vi "pic-labview.vi"() -> ()   [LabVIEW 2020]
uses:
  <vilib>/Instr/_visa.llb/VISA Configure Serial Port (Instr).vi
  <vilib>/ErrorRing/Error Ring.xnode
panel:
  out "error out":errorcluster
  out "reference out":refnum<visa-resource-name>
  in  "Boolean 4":bool
  in  "Boolean 3":bool
  in  "Boolean 2":bool
  in  "Boolean":bool
  out "Thermometer":i32(slide) scale=0.0..1023.0
  out "value":i32
  out "read buffer":string
  in  "Puerto Serial":refnum<visa-resource-name>
  in  "stop":bool
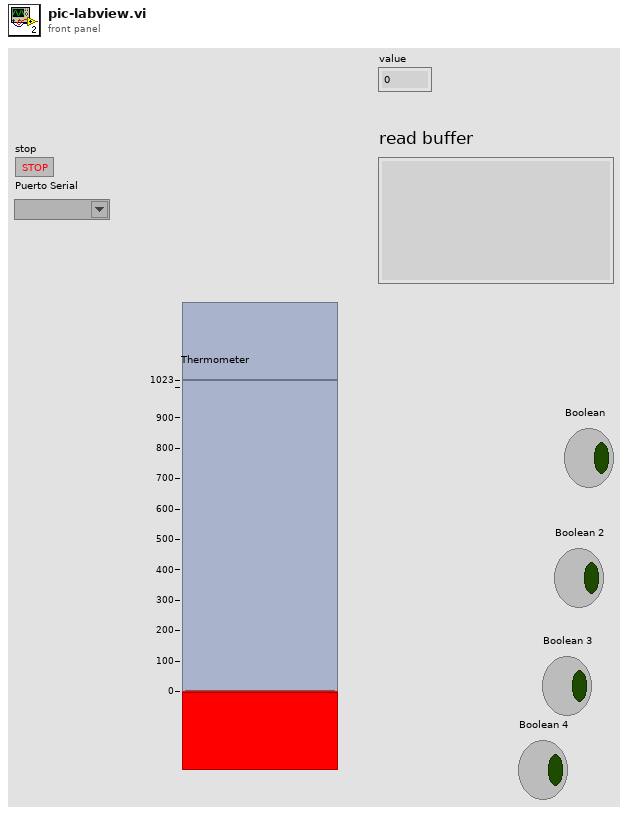
[diagram p1: front panel]
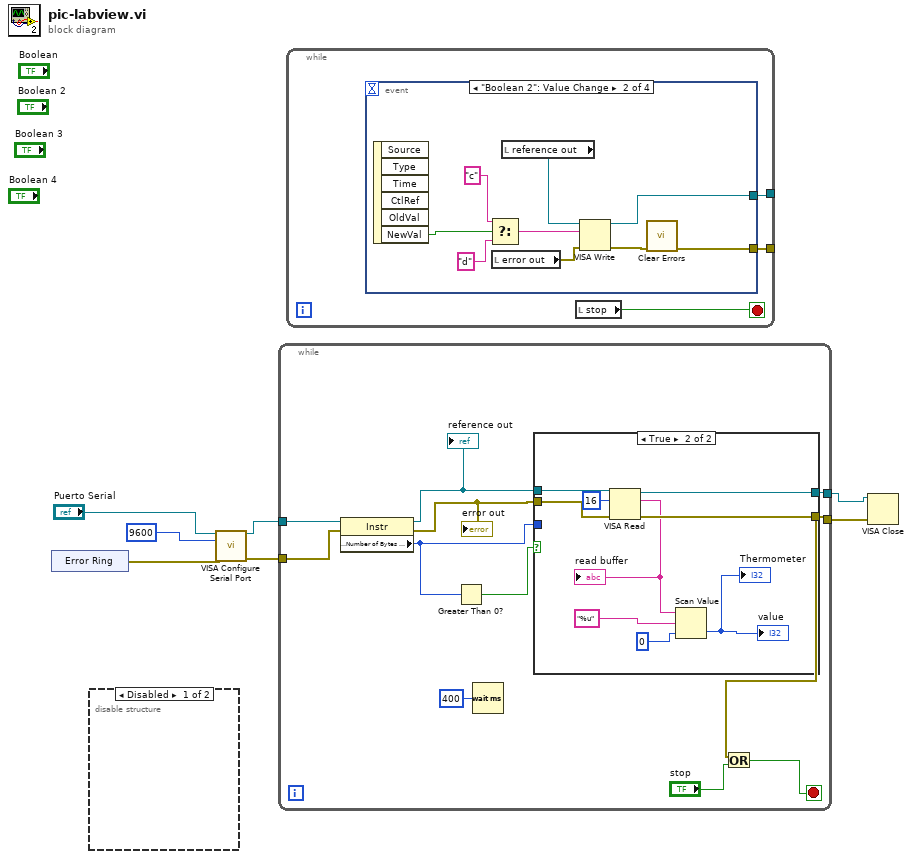
[diagram p0: block diagram]
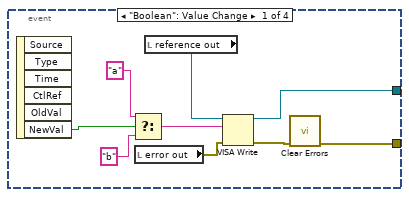
[diagram p2: hidden frame]
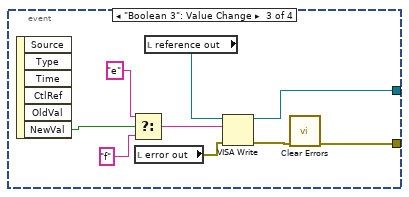
[diagram p3: hidden frame]
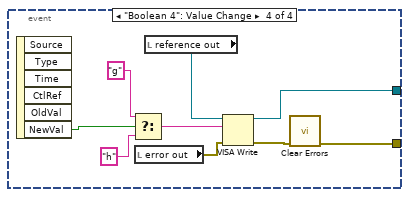
[diagram p4: hidden frame]
diagram:
  n1 = xnode "Error Ring"() -> ("error out"=w6:errorcluster)
  n2 = disable-structure shown="Disabled" {
    frame Disabled {
    }
    frame Enabled {
    }
  }
  n3 = call-poly "VISA Configure Serial Port"("VISA resource name"="Puerto Serial", "baud rate (9600)"=u32 9600, "error in (no error)"=w6) -> ("VISA resource name out"=w4:refnum<visa-resource-name>, "error out"=w3:errorcluster)  [unwired: 11 in]
  n4 = while {
    tunnel: w4 -> [w16]
    tunnel: w3 -> [w15]
    tunnel: [w10] -> w2
    tunnel: [w9] -> w1
    stop <- w18 stop-if-true
    n5 = property class="Instr"(reference=w16, error in=w15) -> (reference out=w13:refnum<visa-resource-name>, error out=w12:errorcluster, "Serial Settings:Number of Bytes at Serial Port"=w11:u32)
    "reference out" <- w13
    "error out" <- w12
    n6 = Greater Than 0?(x=w11) -> (x > 0?=w14:bool)
    n7 = Wait (ms)(milliseconds to wait=u32 400) -> ()  [unwired: 1 out]
    n8 = case shown="True" w14 {
      tunnel: w13 -> [w20 w29]
      tunnel: w12 -> [w19 w28]
      tunnel: w11 -> [_ _]
      tunnel: [w20 w27] -> w10
      tunnel: [w19 w26] -> w9
      frame False {
      }
      frame True {
        n9 = VISA Read(VISA resource name=w29, byte count=u32 16, error in (no error)=w28) -> (VISA resource name out=w27:refnum<visa-resource-name>, read buffer=w25:string, error out=w26:errorcluster)  [unwired: 1 out]
        "read buffer" <- w25
        n10 = Scan Value(string=w25, format string="%u", default (0 dbl)=0) -> (value=→"value" →"Thermometer":i32)  [unwired: 1 out]
      }
    }
    n11 = Or(x=w9, y="stop") -> (x .or. y?=w18:bool)
  }
  n12 = while {
    tunnel: [w32] -> _
    tunnel: [w31] -> _
    stop <- w30 stop-if-true
    n13 = event shown="[1] \"Boolean 2\": Value Change" {
      selector: _ -> [_ _ _ _]
      dyn-events: _ -> [_ _ _ _]
      timeout: _ -> [_ _ _ _]
      tunnel: [w34 w43 w52 w61] -> w32
      tunnel: [w33 w42 w51 w60] -> w31
      event "Boolean": Value Change {
        n14 = event-data() -> ("NewVal"=w41:bool)  [unwired: 1 in, 5 out]
        n15 = Select(t="a", s=w41, f="b") -> (s? t:f=w38:string)
        n16 = local read "error out"() -> (w36:errorcluster)
        n17 = local read "reference out"() -> (w37:refnum<visa-resource-name>)
        n18 = VISA Write(VISA resource name=w37, write buffer=w38, error in (no error)=w36) -> (VISA resource name out=w33:refnum<visa-resource-name>, error out=w35:errorcluster)  [unwired: 1 out]
        n19 = call <vilib>:"Clear Errors.vi"("error in (no error)"=w35) -> ("error out"=w34:errorcluster)  [unwired: 5 in, 1 out]
      }
      event "Boolean 2": Value Change {
        n20 = event-data() -> ("NewVal"=w50:bool)  [unwired: 1 in, 5 out]
        n21 = Select(t="c", s=w50, f="d") -> (s? t:f=w47:string)
        n22 = local read "error out"() -> (w45:errorcluster)
        n23 = local read "reference out"() -> (w46:refnum<visa-resource-name>)
        n24 = VISA Write(VISA resource name=w46, write buffer=w47, error in (no error)=w45) -> (VISA resource name out=w42:refnum<visa-resource-name>, error out=w44:errorcluster)  [unwired: 1 out]
        n25 = call <vilib>:"Clear Errors.vi"("error in (no error)"=w44) -> ("error out"=w43:errorcluster)  [unwired: 5 in, 1 out]
      }
      event "Boolean 3": Value Change {
        n26 = event-data() -> ("NewVal"=w59:bool)  [unwired: 1 in, 5 out]
        n27 = Select(t="e", s=w59, f="f") -> (s? t:f=w56:string)
        n28 = local read "error out"() -> (w54:errorcluster)
        n29 = local read "reference out"() -> (w55:refnum<visa-resource-name>)
        n30 = VISA Write(VISA resource name=w55, write buffer=w56, error in (no error)=w54) -> (VISA resource name out=w51:refnum<visa-resource-name>, error out=w53:errorcluster)  [unwired: 1 out]
        n31 = call <vilib>:"Clear Errors.vi"("error in (no error)"=w53) -> ("error out"=w52:errorcluster)  [unwired: 5 in, 1 out]
      }
      event "Boolean 4": Value Change {
        n32 = event-data() -> ("NewVal"=w68:bool)  [unwired: 1 in, 5 out]
        n33 = Select(t="g", s=w68, f="h") -> (s? t:f=w65:string)
        n34 = local read "error out"() -> (w63:errorcluster)
        n35 = local read "reference out"() -> (w64:refnum<visa-resource-name>)
        n36 = VISA Write(VISA resource name=w64, write buffer=w65, error in (no error)=w63) -> (VISA resource name out=w60:refnum<visa-resource-name>, error out=w62:errorcluster)  [unwired: 1 out]
        n37 = call <vilib>:"Clear Errors.vi"("error in (no error)"=w62) -> ("error out"=w61:errorcluster)  [unwired: 5 in, 1 out]
      }
    }
    n38 = local read "stop"() -> (w30:bool)
  }
  n39 = VISA Close(VISA resource name=w2, error in (no error)=w1) -> ()  [unwired: 1 out]
